vi "picos.set.vi"(8 "error in (no error)":errorcluster, 10 "picos":i64, 11 "endingTimestamp in":refnum<class "endingTimestamp.lvclass">) -> (0 "error out":errorcluster, 3 "endingTimestamp out":refnum<class "endingTimestamp.lvclass">)   [LabVIEW 2020, in "nominal types.lvlib" / "timestampManifest.lvlib" / "endingTimestamp.lvclass"]
uses:
  endingTimestamp.lvclass
  endingTimestamp.lvclass/endingTimestamp.ctl
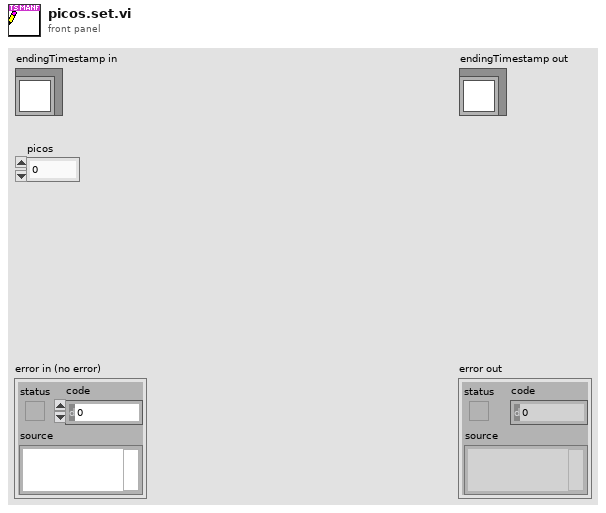
[diagram p1: front panel]
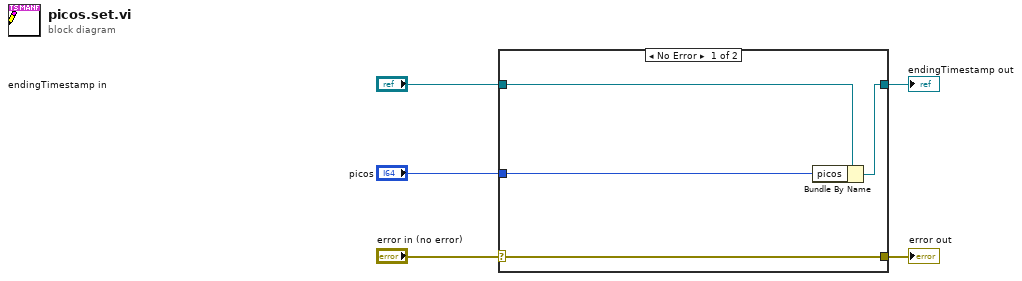
[diagram p0: block diagram]
diagram:
  n1 = case shown="No Error" "error in (no error)" {
    selector: "error in (no error)" -> [w9 w10]
    tunnel: [w9 w10] -> w4
    tunnel: [w7 w11] -> w2
    tunnel: "endingTimestamp in" -> [w8 w11]
    tunnel: "picos" -> [w6 _]
    frame No Error {
      n2 = Bundle By Name(cluster=w8, "picos"=w6) -> (w7:refnum<class "endingTimestamp.lvclass">)
    }
    frame Error {
    }
  }
  "error out" <- w4
  "endingTimestamp out" <- w2
